vi "AprilTag Get Next State.vi"(11 "AprilTag Main Cluster in":T2) -> (1 "Next State":T1, 3 "AprilTag Main Cluster out":T2)   [LabVIEW 2025]
uses:
  AprialTag Main Cluster.ctl
  AprialTag States.ctl
  <vilib>/vision/Image Controls.llb/IMAQ Image.ctl
  <vilib>/vision/Calibration.llb/Internal Parameters.ctl
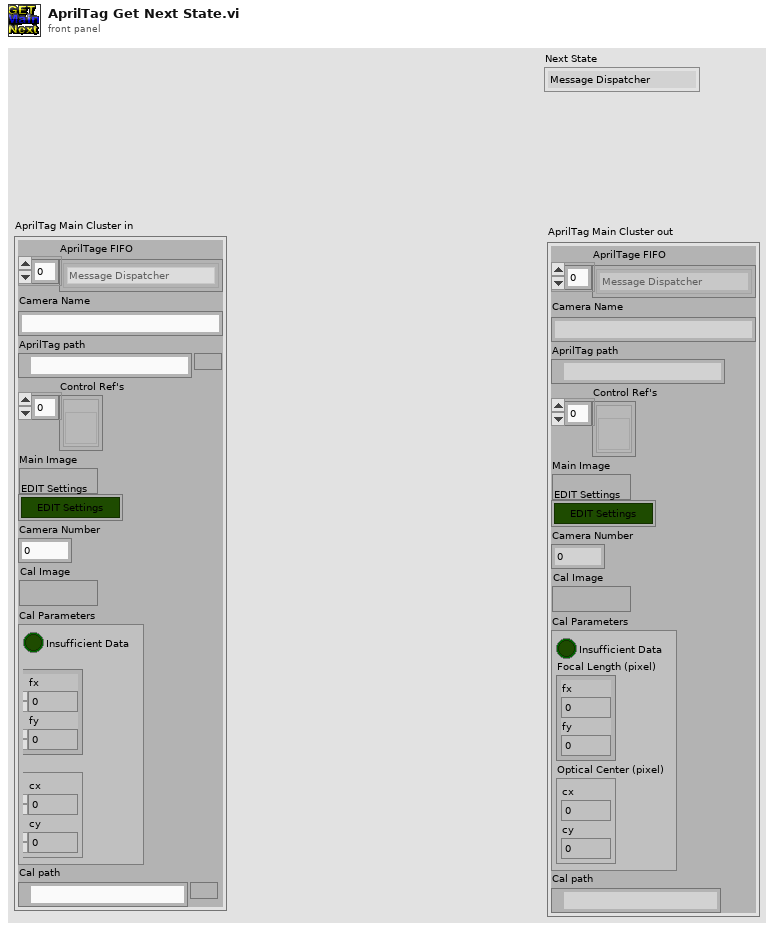
[diagram p1: front panel]
types:
  T1 = typedef "AprialTag States.ctl" = enum16{"Message Dispatcher", "INI", "Open", "Save", "Exit"}
  T2 = typedef "AprialTag Main Cluster.ctl" = cluster{"AprilTage FIFO":T1[], "Camera Name":string, "AprilTag path":path, "Control Ref's":refnum<vi>[], "Main Image":T3, "EDIT Settings":bool, "Camera Number":dbl, "Cal Image":T3, "Cal Parameters":T4, "Cal path":path}
  T3 = typedef "IMAQ Image.ctl" = refnum<image>
  T4 = typedef "Internal Parameters.ctl" = cluster{"Insufficient Data":bool, "Focal Length (pixel)":cluster{"fx":sgl, "fy":sgl}, "Optical Center (pixel)":cluster{"cx":sgl, "cy":sgl}}
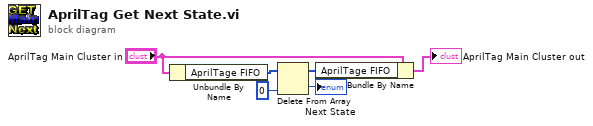
[diagram p0: block diagram]
diagram:
  n1 = Unbundle By Name("AprilTag Main Cluster in") -> ("AprilTage FIFO"=w6:T1[])
  n2 = Delete From Array(array=w6, index=0) -> (deleted portion=→"Next State":T1, array with subset deleted=w4:T1[])  [unwired: 1 in]
  n3 = Bundle By Name(cluster="AprilTag Main Cluster in", "AprilTage FIFO"=w4) -> (→"AprilTag Main Cluster out":T2)
